vi "SSL Write.vi"(8 "Error In":errorcluster, 10 "Input Message":string="Hi, this is Server replying !!!", 11 "SSL Stream":refnum<k24>) -> (0 "Error Out":errorcluster)   [LabVIEW 2014, in "SSL Lib.lvlib"]
doc: "VI Function: This VI writes the data to the client over SSL Stream.\n\nVI Version: 1.0\n\nVI Author: Runjhun Agarwal"
uses:
  <userlib>/SSL Library/SSL Lib.lvlib
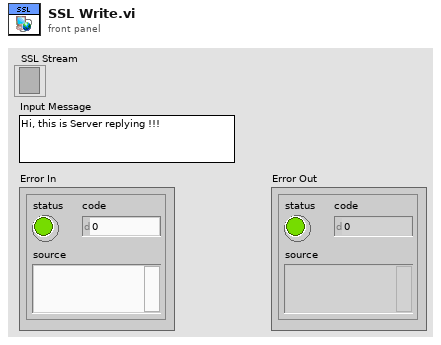
[diagram p1: front panel]
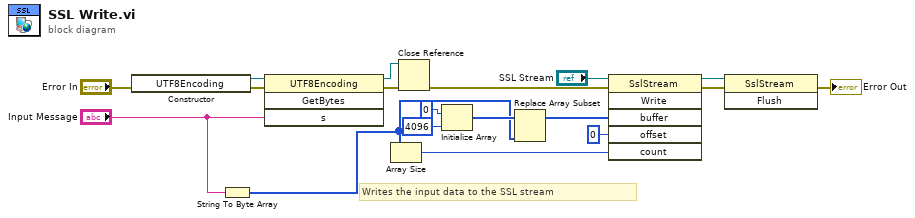
[diagram p0: block diagram]
diagram:
  # "Writes the input data to the SSL stream"
  n1 = constructor class="UTF8Encoding"(error in="Error In") -> (reference out=w16:refnum<k24>, error out=w18:errorcluster)  [unwired: 2 in, 1 out]
  n2 = String To Byte Array(string="Input Message") -> (unsigned byte array=w1:u8[])
  n3 = invoke class="UTF8Encoding" method="GetBytes"(reference=w16, error in=w18, "s"="Input Message") -> (reference out=w14:refnum<k24>, error out=w15:errorcluster)  [unwired: 1 in, 2 out]
  n4 = Array Size(array=w1) -> (size(s)=w11:i32)
  n5 = Close Reference(reference=w14, error in (no error)=w15) -> (error out=w4:errorcluster)
  n6 = Initialize Array(u8 0, 4096 ("dimension size")) -> (w9:u8[])
  n7 = Replace Array Subset(array=w9, new element=w1) -> (w8:u8[])  [unwired: 1 in]
  n8 = invoke class="SslStream" method="Write"(reference="SSL Stream", error in=w4, "buffer"=w8, "offset"=0, "count"=w11) -> (reference out=w7:refnum<k24>, error out=w6:errorcluster)  [unwired: 1 in, 4 out]
  n9 = invoke class="SslStream" method="Flush"(reference=w7, error in=w6) -> (error out=→"Error Out":errorcluster)  [unwired: 1 in, 2 out]
